vi "GetMatlabDefaultValue.vi"(10 "From Value Type":variant, 11 "MatlabType":T1) -> (3 "Default Value":variant)   [LabVIEW 2017]
uses:
  Types/MatlabDataType.ctl
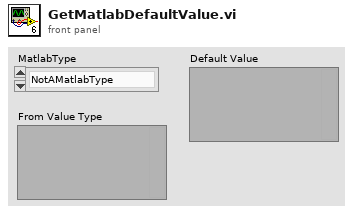
[diagram p1: front panel]
types:
  T1 = typedef "MatlabDataType.ctl" = enum16{"NotAMatlabType", "Real", "Complex", "String", "Boolean"}
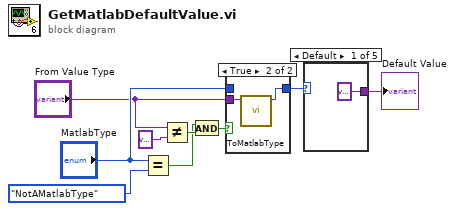
[diagram p0: block diagram]
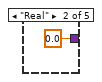
[diagram p3: hidden frame]
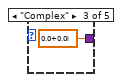
[diagram p4: hidden frame]
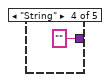
[diagram p5: hidden frame]
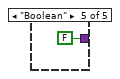
[diagram p6: hidden frame]
diagram:
  n1 = Equal?(x="MatlabType", y=MatlabDataType."NotAMatlabType" ("MatlabType")) -> (x = y?=w5:bool)
  n2 = Not Equal?(x="From Value Type", y=variant ("From Value Type")) -> (x != y?=w6:bool)
  n3 = And(x=w5, y=w6) -> (x .and. y?=w4:bool)
  n4 = case shown="True" w4 {
    tunnel: "MatlabType" -> [w10 _]
    tunnel: [w10 w11] -> w2
    tunnel: "From Value Type" -> [_ w12]
    frame False {
    }
    frame True {
      n5 = call "ToMatlabType.vi"("Value"=w12) -> ("MatlabType"=w11:T1)  [unwired: 7 in, 3 out]
    }
  }
  n6 = case shown="Default" w2 {
    tunnel: [variant 0.0 cdb 0.0+0.0i "" FALSE] -> w9
    frame Default {
    }
    frame "Real" {
    }
    frame "Complex" {
    }
    frame "String" {
    }
    frame "Boolean" {
    }
  }
  "Default Value" <- w9
